vi "Any_Beep.vi"(0 "Length":T1(ring), 4 "Note":T2(ring), 7 "Keithley 2400 (old)":refnum<visa-resource-name>="GPIB0::22::INSTR") -> (3 "Keithley 2400 (old) 2":refnum<visa-resource-name>="GPIB0::22::INSTR")   [LabVIEW 2018]
uses:
  <instrlib>/Keithley 24XX/Keithley 24XX.lvlib
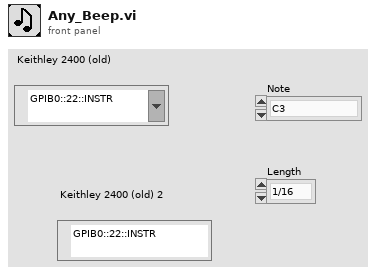
[diagram p1: front panel]
types:
  T1 = enum16{"1/16", "1/8", "1/4", "1/3", "1/2", "1", "3/4", "3/8"}
  T2 = enum16{"C3", "C3#", "D3", "D3#", "E3", "F3", "F3#", "G3", "G3#", "A3", "A3#", "B3", "C4", "C4#", "D4", "D4#", "E4", "F4", "F4#", "G4", "G4#", "A4", "A4#", "B4", "C5"}
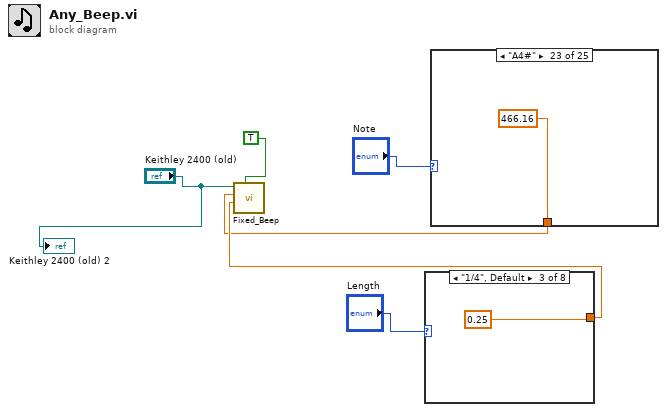
[diagram p0: block diagram]
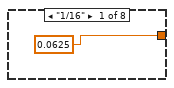
[diagram p2: hidden frame]
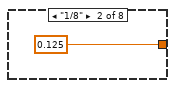
[diagram p3: hidden frame]
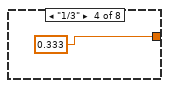
[diagram p4: hidden frame]
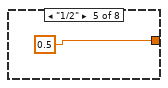
[diagram p5: hidden frame]
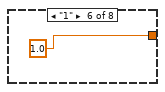
[diagram p6: hidden frame]
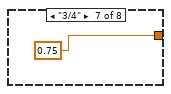
[diagram p7: hidden frame]
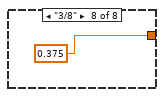
[diagram p8: hidden frame]
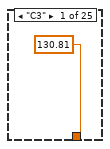
[diagram p9: hidden frame]
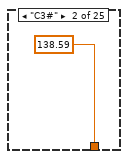
[diagram p10: hidden frame]
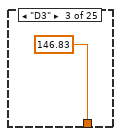
[diagram p11: hidden frame]
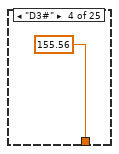
[diagram p12: hidden frame]
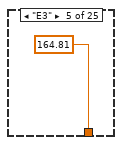
[diagram p13: hidden frame]
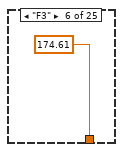
[diagram p14: hidden frame]
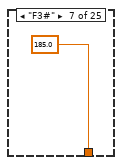
[diagram p15: hidden frame]
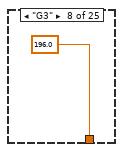
[diagram p16: hidden frame]
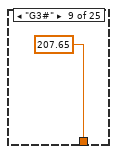
[diagram p17: hidden frame]
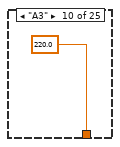
[diagram p18: hidden frame]
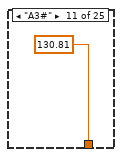
[diagram p19: hidden frame]
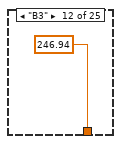
[diagram p20: hidden frame]
diagram:
  n1 = case shown="\"1/4\", Default" "Length" {
    tunnel: [0.0625 0.125 0.25 0.333 0.5 1.0 0.75 0.375] -> w3
    frame "1/16" {
    }
    frame "1/8" {
    }
    frame "1/4", Default {
    }
    frame "1/3" {
    }
    frame "1/2" {
    }
    frame "1" {
    }
    frame "3/4" {
    }
    frame "3/8" {
    }
  }
  n2 = case shown="\"A4#\"" "Note" {
    tunnel: [130.81 138.59 146.83 155.56 164.81 174.61 185.0 196.0 207.65 220.0 130.81 246.94 261.63 277.18 293.66 311.13 329.63 349.23 369.99 392.0 415.3 440.0 466.16 493.88 523.25] -> w2
    frame "C3" {
    }
    frame "C3#" {
    }
    frame "D3" {
    }
    frame "D3#" {
    }
    frame "E3" {
    }
    frame "F3" {
    }
    frame "F3#" {
    }
    frame "G3" {
    }
    frame "G3#" {
    }
    frame "A3" {
    }
    frame "A3#" {
    }
    frame "B3" {
    }
    frame "C4", Default {
    }
    frame "C4#" {
    }
    frame "D4" {
    }
    frame "D4#" {
    }
    frame "E4" {
    }
    frame "F4" {
    }
    frame "F4#" {
    }
    frame "G4" {
    }
    frame "G4#" {
    }
    frame "A4" {
    }
    frame "A4#" {
    }
    frame "B4" {
    }
    frame "C5" {
    }
  }
  n3 = call "Fixed_Beep.vi"("Enable Beep (F)"=TRUE, "Beep Duration (.25 s)"=w3, "Beep Frequency (300)"=w2, "VISA resource name"="Keithley 2400 (old)") -> ()  [unwired: 6 in, 2 out]
  "Keithley 2400 (old) 2" <- "Keithley 2400 (old)"
